vi "Test_StandardLogic_WriteTrue_TerminalEnabled.vi"(8 "error in (no error)":errorcluster, 11 "TestCase in":refnum<class "TestTerminalEnabledStateBinding.lvclass">) -> (0 "error out":errorcluster, 3 "TestCase out":refnum<class "TestTerminalEnabledStateBinding.lvclass">)   [LabVIEW 2017, in "TestTerminalEnabledStateBinding.lvclass"]
uses:
  TestTerminalEnabledStateBinding.lvclass
  Source/Concrete/TerminalEnabledStateBinding/TerminalEnabledStateBinding.lvclass
  C:/Git/composed-transport/Source/ITransport/ITransport.lvclass
  Source/ITransport/ITransport.lvclass
panel:
  in  "Numeric":i32
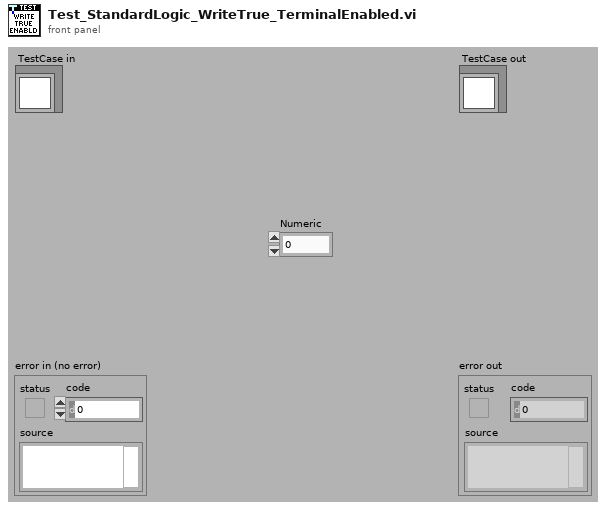
[diagram p1: front panel]
types:
  T1 = enum8{"Enabled", "Disabled", "Disabled and Grayed Out"}
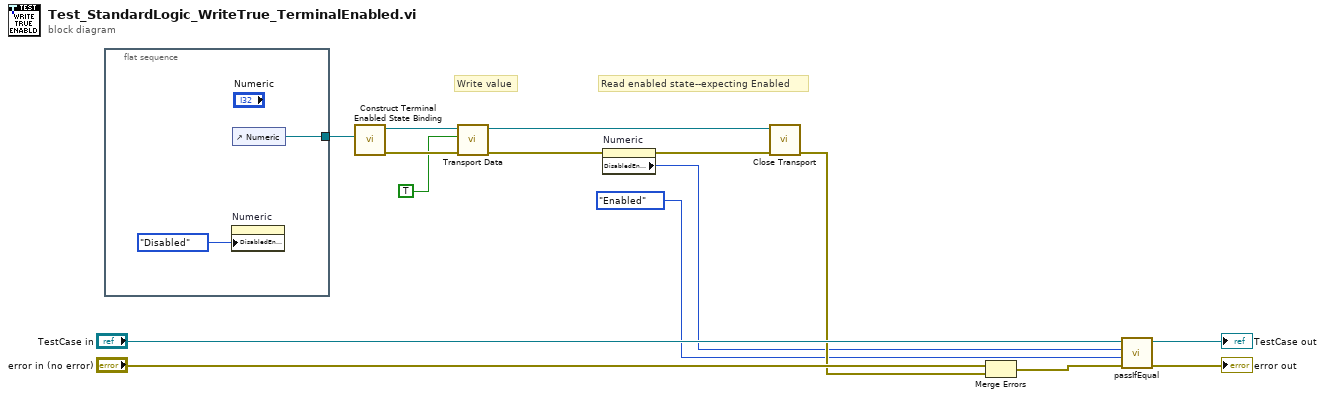
[diagram p0: block diagram]
diagram:
  # "Read enabled state--expecting Enabled"
  # "Write value"
  n1 = flat-sequence {
    tunnel: [w17] -> w6
    frame #0 {
      n2 = property on="Numeric" class="DigNum (strict)"("DisabledEnum"=T1."Disabled" ("Disabled")) -> ()  [unwired: 2 in, 2 out]
      n3 = control-ref of="Numeric"() -> (w17:refnum<vi>)
    }
  }
  n4 = call "Construct Terminal Enabled State Binding.vi"("Control"=w6) -> ("error out"=w9:errorcluster, "TerminalEnabledStateBinding"=w11:refnum<class "TerminalEnabledStateBinding.lvclass">)  [unwired: 9 in]
  n5 = call "Transport Data.vi"("error in (no error)"=w9, "Value"=TRUE, "ITransport in"=w11) -> ("error out"=w5:errorcluster, "ITransport out"=w7:refnum<class "TerminalEnabledStateBinding.lvclass">)  [unwired: 7 in]
  n6 = property on="Numeric" class="DigNum (strict)"(error in=w5) -> (error out=w4:errorcluster, "DisabledEnum"=w2:T1)  [unwired: 1 in, 1 out]
  n7 = call-dynamic "Close Transport.vi"("error in (no error)"=w4, "ITransport in"=w7) -> ("error out"=w3:errorcluster)  [unwired: 9 in]
  n8 = Merge Errors("error in (no error)", w3) -> (w10:errorcluster)
  n9 = call-dynamic "passIfEqual.vi"("error in (no error)"=w10, "y"=T1."Enabled" ("Disabled"), "x"=w2, "TestCase in"="TestCase in") -> ("error out"=→"error out":errorcluster, "TestCase out"=→"TestCase out":refnum<class "TestTerminalEnabledStateBinding.lvclass">)  [unwired: 6 in]
